vi "Configure Spectrum Emission Mask (Offset Setup).vi"(0 "VISA resource name":refnum<visa-resource-name>, 5 "SEM Page Number (1)":i32=1 min=1 max=2, 7 "SEM Offset":i32[](array[ring]) items=["Off", "On"], 11 "error in (no error)":errorcluster) -> (4 "VISA resource name out":refnum<visa-resource-name>, 15 "error out":errorcluster)   [LabVIEW 2020, in "Anritsu Signal Analyzer Series.lvlib"]
doc: "Configures the offset Limit for SEM measurement"
uses:
  Anritsu Signal Analyzer Series.lvlib
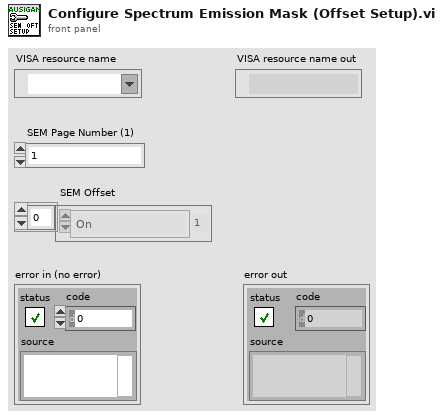
[diagram p1: front panel]
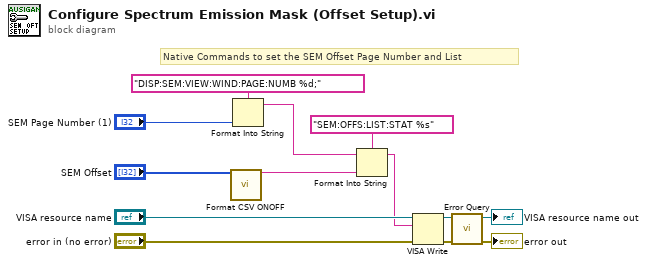
[diagram p0: block diagram]
diagram:
  # "Native Commands to set the SEM Offset Page Number and List"
  n1 = call "Format CSV ONOFF.vi"("Data_In"="SEM Offset") -> ("Data_out"=w4:string)  [unwired: 14 in]
  n2 = Format Into String(format string="DISP:SEM:VIEW:WIND:PAGE:NUMB %d;" ("_CommandSet"), "SEM Page Number (1)") -> (resulting string=w5:string)  [unwired: 2 in, 1 out]
  n3 = Format Into String(format string="SEM:OFFS:LIST:STAT %s" ("_CommandSet"), initial string=w5, w4) -> (resulting string=w7:string)  [unwired: 1 in, 1 out]
  n4 = VISA Write(VISA resource name="VISA resource name", write buffer=w7, error in (no error)="error in (no error)") -> (VISA resource name out=w2:refnum<visa-resource-name>, error out=w1:errorcluster)  [unwired: 1 out]
  n5 = call "Error Query.vi"("error in (no error)"=w1, "VISA resource name"=w2) -> ("error out"=→"error out":errorcluster, "VISA resource name out"=→"VISA resource name out":refnum<visa-resource-name>)  [unwired: 6 in, 2 out]
